vi "Read PID Setpoints.vi"(11 "SD Name":string) -> (2 "PID gains":T1, 3 "output range":cluster{"output high":dbl, "output low":dbl})   [LabVIEW 2013]
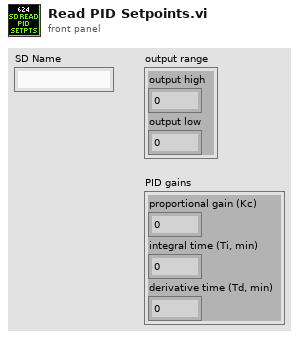
[diagram p1: front panel]
types:
  T1 = cluster{"proportional gain (Kc)":dbl, "integral time (Ti, min)":dbl, "derivative time (Td, min)":dbl}
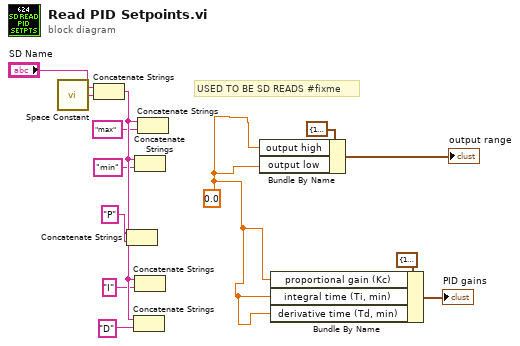
[diagram p0: block diagram]
diagram:
  w1 = 0.0
  # "USED TO BE SD READS #fixme"
  n1 = call <vilib>:"Space Constant.vi"() -> ("String"=w11:string)
  n2 = Concatenate Strings("SD Name", w11) -> (w13:string)
  n3 = Concatenate Strings(w13, "P" ("Name")) -> ()  [unwired: 1 out]
  n4 = Concatenate Strings(w13, "D" ("Name")) -> ()  [unwired: 1 out]
  n5 = Concatenate Strings(w13, "min" ("Name")) -> ()  [unwired: 1 out]
  n6 = Concatenate Strings(w13, "I" ("Name")) -> ()  [unwired: 1 out]
  n7 = Concatenate Strings(w13, "max" ("Name")) -> ()  [unwired: 1 out]
  n8 = Bundle By Name(cluster=cluster{"output high":dbl, "output low":dbl} {"output high"=1.0, "output low"=-1.0} ("output range"), "output high"=w1, "output low"=w1) -> (→"output range":cluster{"output high":dbl, "output low":dbl})
  n9 = Bundle By Name(cluster=T1 {"proportional gain (Kc)"=1.0, "integral time (Ti, min)"=0.0, "derivative time (Td, min)"=0.0} ("PID gains"), "proportional gain (Kc)"=w1, "integral time (Ti, min)"=w1, "derivative time (Td, min)"=w1) -> (→"PID gains":T1)
